vi "servoPulseWidth.vi"() -> ()   [LabVIEW 2020]
panel:
  out "pulse width":u32
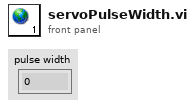
[diagram p1: front panel]
diagram:
